vi "Task by Type.vi"(8 "error in (no error)":errorcluster, 11 "Task Type":string) -> (0 "error out":errorcluster, 3 "Task":refnum<class "Task.lvclass">)   [LabVIEW 2020, in "Volatus.lvlib"]
uses:
  Volatus.lvlib
  Task/Task.lvclass
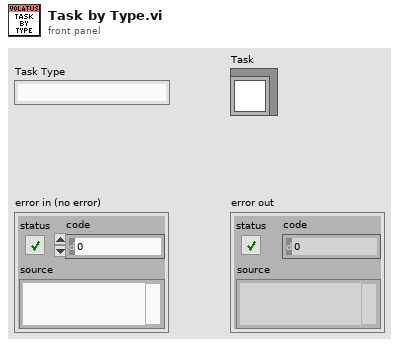
[diagram p1: front panel]
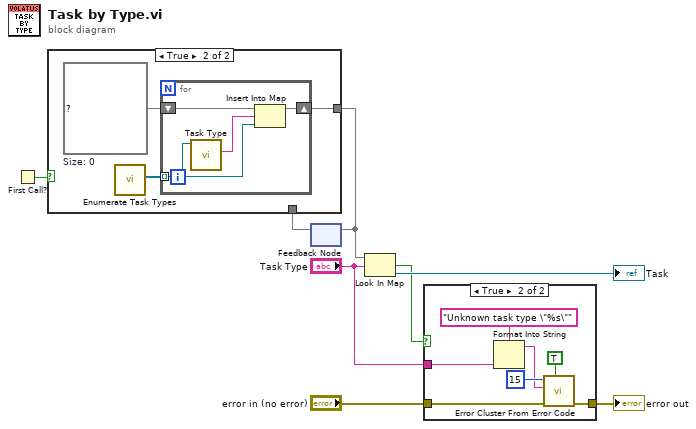
[diagram p0: block diagram]
diagram:
  n1 = First Call?() -> (First Call?: T/F=w8:bool)
  n2 = feedback #1() -> (w7:map{string, refnum<class "Task.lvclass">})  [unwired: 1 in]
  n3 = case shown="True" w8 {
    tunnel: [w9 w10] -> w6
    tunnel: w7 -> [w9 _]
    frame False {
    }
    frame True {
      w11 = map{string, refnum<class "Task.lvclass">} {}  # Size: 0
      n4 = call "Enumerate Task Types.vi"() -> ("All Task Types"=w12:refnum<class "Task.lvclass">[])  [unwired: 11 in]
      n5 = for {
        tunnel: w12 -> [w15] mode=indexing
        shift-right: [w13] -> w10
        shift-left: w11 -> [w16]
        n6 = call-dynamic "Task Type.vi"("Task in"=w15) -> ("Task Type"=w14:string)  [unwired: 10 in]
        n7 = Insert Into Map(map in=w16, key=w14, value=w15) -> (map out=w13:map{string, refnum<class "Task.lvclass">})  [unwired: 2 out]
      }
    }
  }
  n8 = feedback-in #1(w6) -> ()
  n9 = Look In Map(map=w6, key="Task Type") -> (key not found?=w4:bool, value=→"Task":refnum<class "Task.lvclass">)  [unwired: 1 in]
  n10 = case shown="True" w4 {
    tunnel: "Task Type" -> [_ w24]
    tunnel: "error in (no error)" -> [w17 w22]
    tunnel: [w17 w18] -> w1
    frame False {
    }
    frame True {
      n11 = Format Into String(format string="Unknown task type \"%s\"", w24) -> (resulting string=w19:string)  [unwired: 2 in, 1 out]
      n12 = call <vilib>:"Error Cluster From Error Code.vi"("show call chain? (False)"=TRUE, "error in (no error)"=w22, "error message (\"\")"=w19, "error code (0)"=15) -> ("error out"=w18:errorcluster)  [unwired: 5 in]
    }
  }
  "error out" <- w1
